vi "FTW-Test-Expressions-Booleanish.vi"() -> (0 "error out":errorcluster)   [LabVIEW 2015]
uses:
  src/error/FTW-ERR-ExceptionType.ctl
  src/expression/FTW-Expr-BooleanExpressionResult.ctl
  src/error/FTW-ERR-ThrowError.vi
  src/error/FTW-ERR-CallChain.vi
  src/error/FTW-ERR-NoErrorConstant.vi
  src/string/FTW-STR-ReplaceWhitespace.vi
  src/string/FTW-STR-Array-Delimit.vi
  src/error/FTW-ERR-Clear.vi
  src/regex/FTW-Regex-ReplaceAll.vi
  lib/FTW-KernelFilepath.vi
panel:
  out "String":string
  out "Array":string[](array[string])
  out "Results":T3(array[cluster])
  out "Lexicon":string="$test == true || $b == false && $c == false"
  out "Capture Groups":string[](array[string])
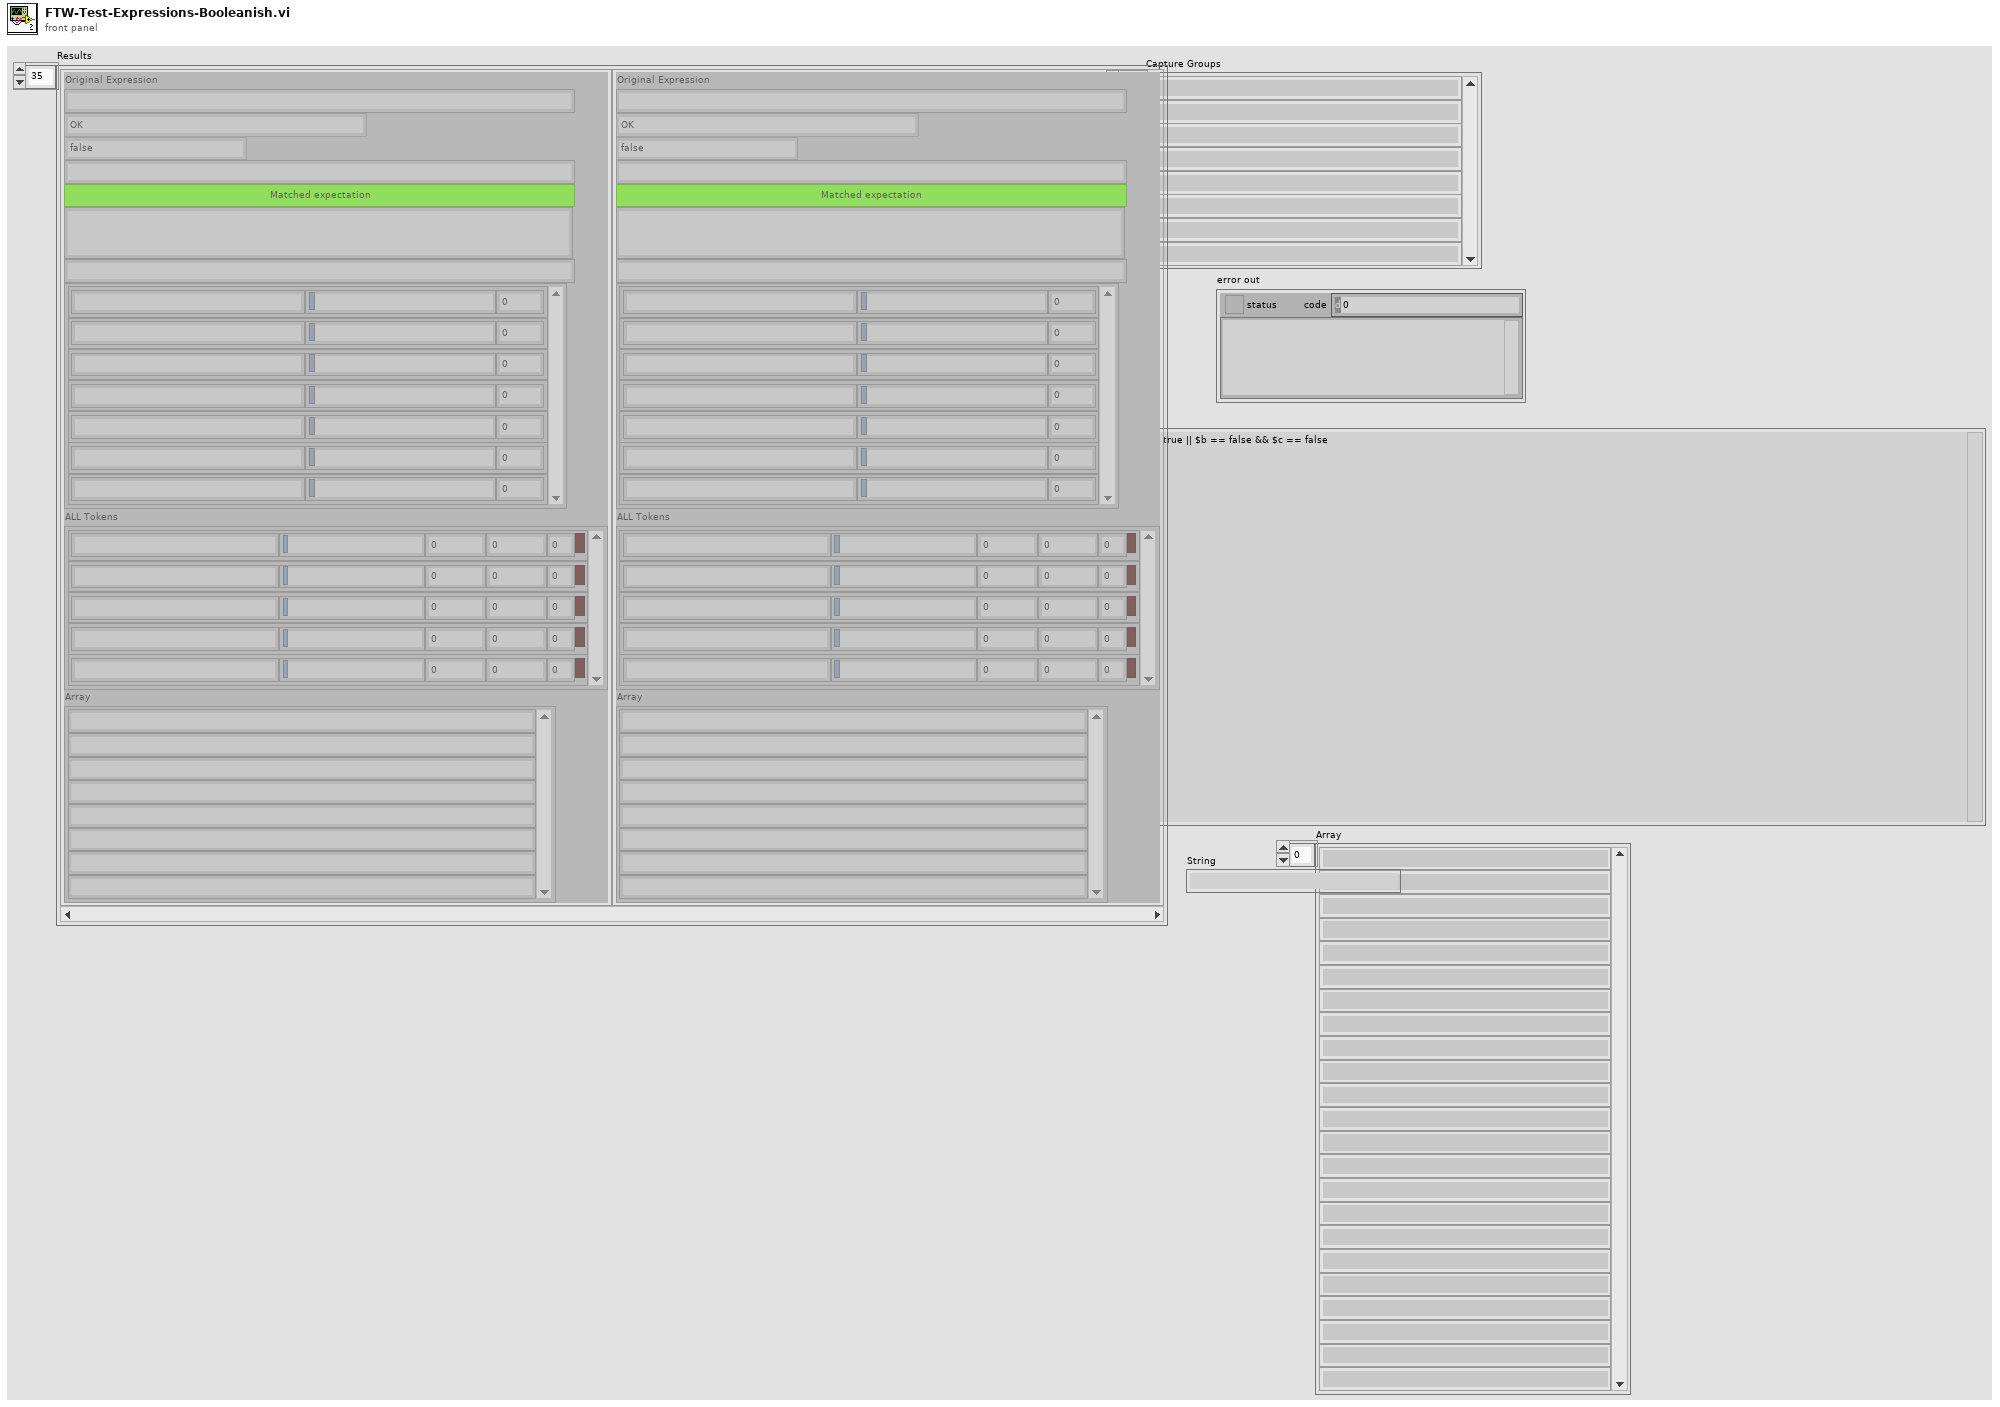
[diagram p1: front panel]
types:
  T1 = typedef "FTW-ERR-ExceptionType.ctl" = enum16{"OK", "Info", "Warning", "Error"}
  T2 = typedef "FTW-Expr-BooleanExpressionResult.ctl" = enum16{"false", "true", "inconclusive"}
  T3 = cluster{"Original Expression":string, "Expression Validity Expectation":T1, "Result":T2, "Expectation":string, "Expectation satisfied?":bool, "Error":string, "Final JSON":string, "Parsed Expression":cluster{string, string, "start_pos":i32}[], "ALL Tokens":cluster{string, string, "prev_pos":i32, "curr_pos":i32, "scope_level":i32, "trimmed?":bool}[], "Array":string[]}[]
  T4 = cluster{"Expression":string, "Expectation":string, "Expression Check":T1, "Value Expectation":T2}[]
  T5 = cluster{"op":cluster{"token":string, "value":string, "subj_start":i32}, "Precedence":i32, "Scope Depth":i32}[]
  T6 = cluster{"token":string, "value":string, "subj_start":i32}[]
  T7 = cluster{"callout_id":i32, "subject_current_pos":i32, "subject_start_match_pos":i32, "cap_top":i32, "cap_last":i32, "patt_pos":i32, "callout_name_index":i32, "callout_name_length":i32}[]
  T8 = cluster{"Text":string, "Expression":string, "Previous Subject Position":i32}
  T9 = cluster{"Text":string, "Expression":string, "Previous Subject Position":i32}[]
  T10 = cluster{cluster{"Text":string, "Expression":string, "Previous Subject Position":i32}, "Precedence":i32, i32}
  T11 = cluster{"op":cluster{"token":string, "value":string, "subj_start":i32}, "Precedence":i32, "Scope Depth":i32}
  T12 = cluster{"token":string, "value":string, "subj_start":i32}
  T13 = cluster{cluster{"Text":string, "Expression":string, "Previous Subject Position":i32}, "default value 1":i32, "Current Scope Depth":i32}
  T14 = cluster{"Text":string, "Expression":string, "subject_current_pos":i32, "Previous Subject Position":i32, "Current Scope Depth":i32, bool}
  T15 = typedef "FTW-JSON-Type.ctl" = enum8{"Not Found", "Object", "Array", "String", "Number", "Boolean", "null"}
  T16 = cluster{"Expression":string, "Expression Check":T1, "Result":T2, "Expectation":string, bool, "source":string, "JSON String (UTF-8)":string, "Reverse Polish Notation Token Stack":cluster{"token":string, "value":string, "subj_start":i32}[], cluster{"Text":string, "Expression":string, "subject_current_pos":i32, "Previous Subject Position":i32, "Current Scope Depth":i32, bool}[], "Try Paths":string[]}
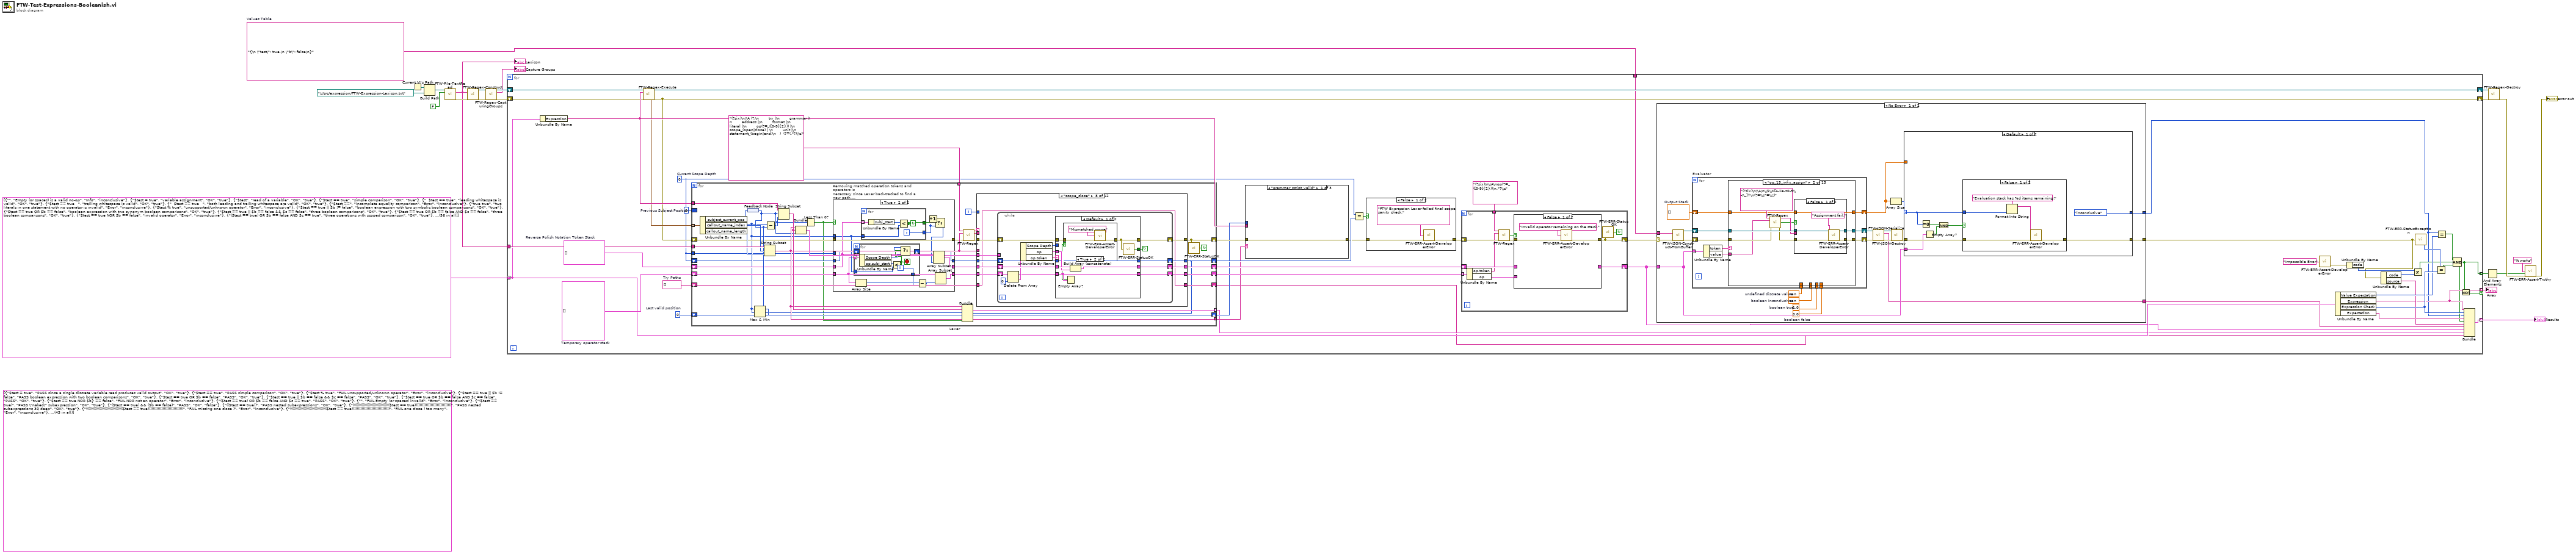
[diagram p0: block diagram]
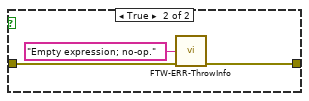
[diagram p2: hidden frame]
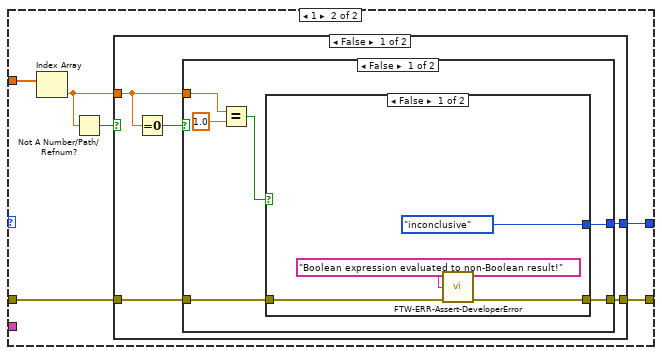
[diagram p3: hidden frame]
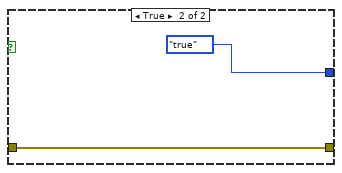
[diagram p4: hidden frame]
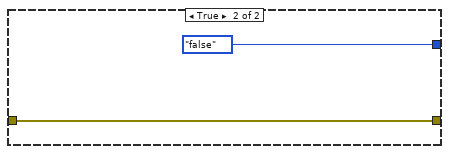
[diagram p5: hidden frame]
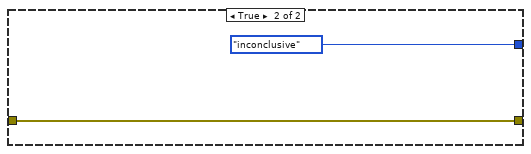
[diagram p6: hidden frame]
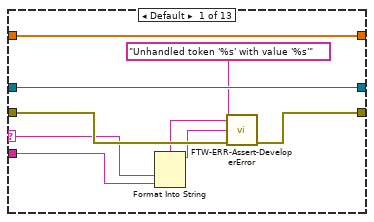
[diagram p7: hidden frame]
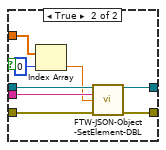
[diagram p8: hidden frame]
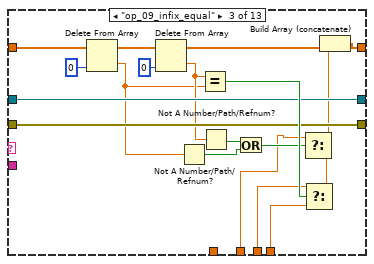
[diagram p9: hidden frame]
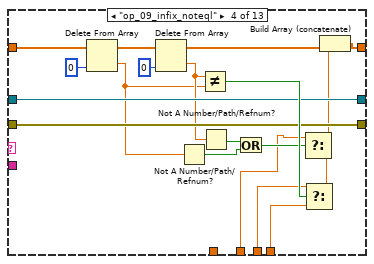
[diagram p10: hidden frame]
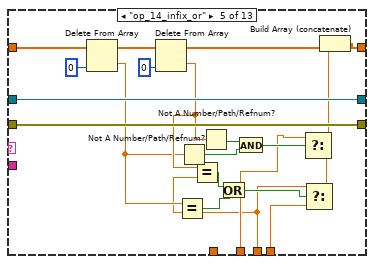
[diagram p11: hidden frame]
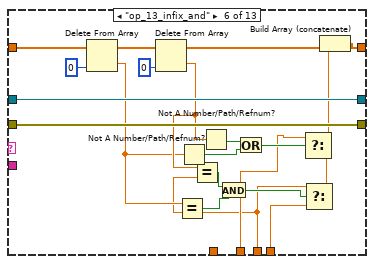
[diagram p12: hidden frame]
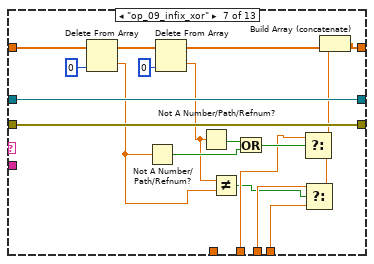
[diagram p13: hidden frame]
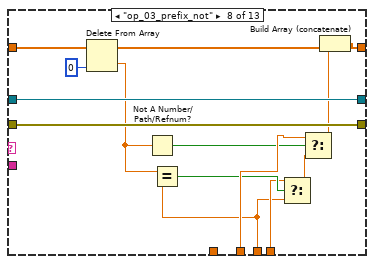
[diagram p14: hidden frame]
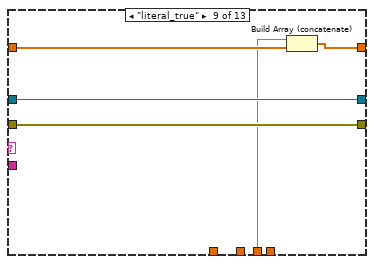
[diagram p15: hidden frame]
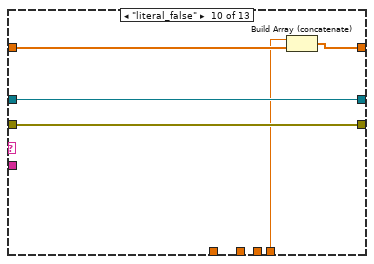
[diagram p16: hidden frame]
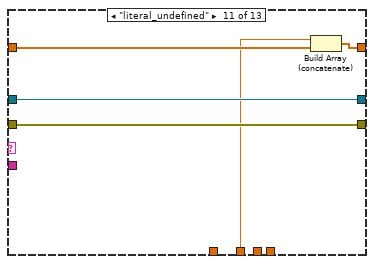
[diagram p17: hidden frame]
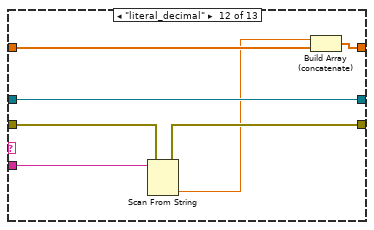
[diagram p18: hidden frame]
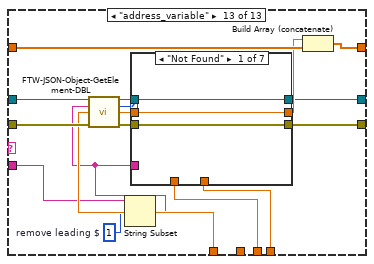
[diagram p19: hidden frame]
diagram:
  (unwired) T4 [{"Expression"="$test = true", "Expectation"="PASS since a single discrete variable read produces valid output", "Expression Check"=enum."OK", "Value Expectation"=enum."true"}, {"Expression"="$test == true", "Expectation"="PASS simple comparison", "Expression Check"=enum."OK", "Value Expectation"=enum."true"}, {"Expression"="$test % true", "Expectation"="FAIL unsupported/unknown operator", "Expression Check"=enum."Error", "Value Expectation"=enum."inconclusive"}, {"Expression"="$test == true || $b != false", "Expectation"="PASS boolean expression with two boolean comparisons", "Expression Check"=enum."OK", "Value Expectation"=enum."true"}, {"Expression"="$test == true OR $b == false", "Expectation"="PASS", "Expression Check"=enum."OK", "Value Expectation"=enum."true"}, {"Expression"="$test == true || $b == false && $c == false", "Expectation"="PASS", "Expression Check"=enum."OK", "Value Expectation"=enum."true"}, {"Expression"="$test == true OR $b == false AND $c == false", "Expectation"="PASS", "Expression Check"=enum."OK", "Value Expectation"=enum."true"}, {"Expression"="$test == true NOR $b} == false", "Expectation"="FAIL NOR not an operator", "Expression Check"=enum."Error", "Value Expectation"=enum."inconclusive"}, {"Expression"="($test == true) OR $b == false AND $c == true", "Expectation"="PASS", "Expression Check"=enum."OK", "Value Expectation"=enum."true"}, {"Expression"="", "Expectation"="FAIL Empty (or spaces) invalid", "Expression Check"=enum."Error", "Value Expectation"=enum."inconclusive"}, {"Expression"="($test == true)", "Expectation"="PASS \"naked\" subexpression", "Expression Check"=enum."OK", "Value Expectation"=enum."true"}, {"Expression"="($test == true) && ($b == false)", "Expectation"="PASS", "Expression Check"=enum."OK", "Value Expectation"=enum."false"}, {"Expression"="(($test == true))", "Expectation"="PASS nested subexpressions", "Expression Check"=enum."OK", "Value Expectation"=enum."true"}, {"Expression"="(((((((((((((((((((((((((((((($test == true))))))))))))))))))))))))))))))", "Expectation"="PASS nested subexpressions 30 deep", "Expression Check"=enum."OK", "Value Expectation"=enum."true"}, {"Expression"="(((((((((((((((((((((((((((((($test == true)))))))))))))))))))))))))))))", "Expectation"="FAIL missing one close )", "Expression Check"=enum."Error", "Value Expectation"=enum."inconclusive"}, {"Expression"="(((((((((((((((((((((((((((((($test == true)))))))))))))))))))))))))))))))", "Expectation"="FAIL one close ) too many", "Expression Check"=enum."Error", "Value Expectation"=enum."inconclusive"}, {"Expression"="true", "Expectation"="PASS plain constant", "Expression Check"=enum."OK", "Value Expectation"=enum."true"}, {"Expression"="False", "Expectation"="PASS plain constant", "Expression Check"=enum."OK", "Value Expectation"=enum."false"}, {"Expression"="ALWAYS AND NEVER", "Expectation"="PASS expression of two boolexpr constants", "Expression Check"=enum."OK", "Value Expectation"=enum."inconclusive"}, {"Expression"="ALWAYS XOR NEVER", "Expectation"="PASS expression of two boolexpr constants", "Expression Check"=enum."OK", "Value Expectation"=enum."inconclusive"}, {"Expression"="(true == true) AND (true EQUALS true) AND (true IS true)", "Expectation"="PASS testing equality operators", "Expression Check"=enum."OK", "Value Expectation"=enum."true"}, {"Expression"="(true != false) AND (true IS NOT false) AND (true <> false)", "Expectation"="PASS testing inequality operators", "Expression Check"=enum."OK", "Value Expectation"=enum."true"}, {"Expression"="(always AND never) XOR (never AND always)", "Expectation"="PASS compound expression of boolexpr constants", "Expression Check"=enum."OK", "Value Expectation"=enum."false"}, {"Expression"="$A==$B", "Expectation"="PASS compare two variables to each other", "Expression Check"=enum."OK", "Value Expectation"=enum."inconclusive"}, {"Expression"="$a!=$b", "Expectation"="PASS since this is a synonym for XOR", "Expression Check"=enum."OK", "Value Expectation"=enum."inconclusive"}, {"Expression"="$A AND $B", "Expectation"="PASS assuming, variables are boolexpr states", "Expression Check"=enum."OK", "Value Expectation"=enum."inconclusive"}, {"Expression"="$a IS true for 3 sec", "Expectation"="SKIP PASS simple timer test", "Expression Check"=enum."OK", "Value Expectation"=enum."inconclusive"}, {"Expression"="$a IS true for 3min", "Expectation"="SKIP PASS no space between timer value and unit", "Expression Check"=enum."OK", "Value Expectation"=enum."inconclusive"}, {"Expression"="$a IS true for 3", "Expectation"="SKIP FAIL no timer units", "Expression Check"=enum."OK", "Value Expectation"=enum."inconclusive"}, {"Expression"="$a IS true   for minute", "Expectation"="SKIP FAIL no timer value", "Expression Check"=enum."OK", "Value Expectation"=enum."inconclusive"}, {"Expression"="$a == true || $b AND $c", "Expectation"="PASS", "Expression Check"=enum."OK", "Value Expectation"=enum."inconclusive"}, {"Expression"="alwaysornever", "Expectation"="FAIL no word boundary on neither operator nor constants", "Expression Check"=enum."OK", "Value Expectation"=enum."inconclusive"}, {"Expression"="always||never", "Expectation"="PASS even though no spaces, the symbolic operator makes a word boundary", "Expression Check"=enum."OK", "Value Expectation"=enum."inconclusive"}, {"Expression"="(($a&&$b) OR ($c&&$d)) AND (($e&&$f) OR ($g&&$h))", "Expectation"="PASS compound expression", "Expression Check"=enum."OK", "Value Expectation"=enum."inconclusive"}, {"Expression"="$a (AND $b)", "Expectation"="FAIL improper placement of parentheses", "Expression Check"=enum."OK", "Value Expectation"=enum."inconclusive"}, {"Expression"="($a)($b)", "Expectation"="FAIL no operator between scopes", "Expression Check"=enum."OK", "Value Expectation"=enum."inconclusive"}, {"Expression"="($a)                   or                 ($b)", "Expectation"="PASS goofy amount of space", "Expression Check"=enum."OK", "Value Expectation"=enum."inconclusive"}, {"Expression"="NOT ALWAYS", "Expectation"="PASS the inversion of a boolexpr constant", "Expression Check"=enum."OK", "Value Expectation"=enum."inconclusive"}, {"Expression"="NOT $a || $b", "Expectation"="PASS even though it could use some parentheses for clarity, this is valid", "Expression Check"=enum."OK", "Value Expectation"=enum."inconclusive"}, {"Expression"="NOT ($a || $b)", "Expectation"="PASS", "Expression Check"=enum."OK", "Value Expectation"=enum."inconclusive"}, {"Expression"="(NOT $a) || $b", "Expectation"="PASS", "Expression Check"=enum."OK", "Value Expectation"=enum."inconclusive"}, {"Expression"="$a && !$b", "Expectation"="PASS", "Expression Check"=enum."OK", "Value Expectation"=enum."inconclusive"}, {"Expression"="IMMEDIATELY", "Expectation"="PASS this is a synonym for ALWAYS", "Expression Check"=enum."OK", "Value Expectation"=enum."inconclusive"}]
  w8 = "{\n \"test\": true,\n \"b\": false\n}"  # Values Table
  n1 = Current VI's Path() -> (path=w18:path)
  n2 = Build Path(base path=w18, name or relative path=path "../../../src/expression/FTW-Expression-Lexicon.txt" ("path")) -> (appended path=w16:path)
  n3 = call "FTW-File-TextRead.vi"("Filepath"=w16, "Create if doesn't exist?"=FALSE) -> ("Text"=w19:string, "error out"=w20:errorcluster)  [unwired: 11 in, 1 out]
  "Lexicon" <- w19
  n4 = call "FTW-Regex-Construct.vi"("Regular Expression"=w19, "error in"=w20) -> ("Regex"=w14:refnum<data-value>, "error out"=w15:errorcluster)  [unwired: 12 in]
  n5 = call "FTW-Regex-CapturingGroups.vi"("Regex"=w14, "error in"=w15) -> ("Regex out"=w22:refnum<data-value>, "Capture Groups"=→"Capture Groups":string[], "error out"=w9:errorcluster)  [unwired: 11 in]
  n6 = for {
    tunnel: w19 -> [w70]
    shift-right: [w55] -> w12
    shift-left: w22 -> [w71]
    tunnel: T4 [{"Expression"="", "Expectation"="Empty (or spaces) is a valid no-op", "Expression Check"=enum."Info", "Value Expectation"=enum."inconclusive"}, {"Expression"="$test = true", "Expectation"="variable assignment", "Expression Check"=enum."OK", "Value Expectation"=enum."true"}, {"Expression"="$test", "Expectation"="read of a variable", "Expression Check"=enum."OK", "Value Expectation"=enum."true"}, {"Expression"="$test == true", "Expectation"="simple comparison", "Expression Check"=enum."OK", "Value Expectation"=enum."true"}, {"Expression"="  $test == true", "Expectation"="leading whitespace is valid", "Expression Check"=enum."OK", "Value Expectation"=enum."true"}, {"Expression"="$test == true   ", "Expectation"="trailing whitespace is valid", "Expression Check"=enum."OK", "Value Expectation"=enum."true"}, {"Expression"="  $test == true   ", "Expectation"="both leading and trailing whitespace are valid", "Expression Check"=enum."OK", "Value Expectation"=enum."true"}, {"Expression"="$test ==", "Expectation"="incomplete equality comparison", "Expression Check"=enum."Error", "Value Expectation"=enum."inconclusive"}, {"Expression"="true true", "Expectation"="two literals in one statement with no operator is invalid", "Expression Check"=enum."Error", "Value Expectation"=enum."inconclusive"}, {"Expression"="$test % true", "Expectation"="unsupported/unknown operator", "Expression Check"=enum."Error", "Value Expectation"=enum."inconclusive"}, {"Expression"="$test == true || $b != false", "Expectation"="boolean expression with two symbolic boolean comparisons", "Expression Check"=enum."OK", "Value Expectation"=enum."true"}, {"Expression"="$test == true OR $b == false", "Expectation"="boolean expression with two synonym boolean comparisons", "Expression Check"=enum."OK", "Value Expectation"=enum."true"}, {"Expression"="$test == true || $b == false && $c == false", "Expectation"="three boolean comparisons", "Expression Check"=enum."OK", "Value Expectation"=enum."true"}, {"Expression"="$test == true OR $b == false AND $c == false", "Expectation"="three boolean comparisons", "Expression Check"=enum."OK", "Value Expectation"=enum."true"}, {"Expression"="$test == true NOR $b == false", "Expectation"="invalid operator", "Expression Check"=enum."Error", "Value Expectation"=enum."inconclusive"}, {"Expression"="($test == true) OR $b == false AND $c == true", "Expectation"="three operations with scoped comparison", "Expression Check"=enum."OK", "Value Expectation"=enum."true"}, {"Expression"="$test OR ($test == false)", "Expectation"="variable comparison with subexpression", "Expression Check"=enum."OK", "Value Expectation"=enum."true"}, {"Expression"="($test == true)", "Expectation"="superfluous subexpression", "Expression Check"=enum."OK", "Value Expectation"=enum."true"}, {"Expression"="($test == true) && ($b == false)", "Expectation"="operation on two subexpressions", "Expression Check"=enum."OK", "Value Expectation"=enum."true"}, {"Expression"="(($test == true))", "Expectation"="nested subexpressions", "Expression Check"=enum."OK", "Value Expectation"=enum."true"}, {"Expression"="(((((((((((((((((((((((((((((($test == true))))))))))))))))))))))))))))))", "Expectation"="PASS nested subexpressions 30 deep", "Expression Check"=enum."OK", "Value Expectation"=enum."true"}, {"Expression"="(((((((((((((((((((((((((((((($test == true)))))))))))))))))))))))))))))", "Expectation"="missing one close )", "Expression Check"=enum."Error", "Value Expectation"=enum."inconclusive"}, {"Expression"="(((((((((((((((((((((((((((((($test == true)))))))))))))))))))))))))))))))", "Expectation"="one close ) too many", "Expression Check"=enum."Error", "Value Expectation"=enum."inconclusive"}, {"Expression"="true", "Expectation"="plain constant", "Expression Check"=enum."OK", "Value Expectation"=enum."true"}, {"Expression"="False", "Expectation"="plain constant", "Expression Check"=enum."OK", "Value Expectation"=enum."false"}, {"Expression"="true XOR false", "Expectation"="expression of two boolexpr constants", "Expression Check"=enum."OK", "Value Expectation"=enum."true"}, {"Expression"="(true == true) AND (true EQUALS true) AND (true IS true)", "Expectation"="testing equality operators", "Expression Check"=enum."OK", "Value Expectation"=enum."true"}, {"Expression"="(true != false) AND (true IS NOT false) AND (true <> false)", "Expectation"="testing inequality operators", "Expression Check"=enum."OK", "Value Expectation"=enum."true"}, {"Expression"="(true AND false) XOR (false AND true)", "Expectation"="compound expression of boolexpr constants", "Expression Check"=enum."OK", "Value Expectation"=enum."false"}, {"Expression"="$A==$B", "Expectation"="compare two variables to each other", "Expression Check"=enum."OK", "Value Expectation"=enum."inconclusive"}, {"Expression"="$a!=$b", "Expectation"="synonym for XOR", "Expression Check"=enum."OK", "Value Expectation"=enum."inconclusive"}, {"Expression"="$A AND $B", "Expectation"="AND two variables", "Expression Check"=enum."OK", "Value Expectation"=enum."inconclusive"}, {"Expression"="$test == ture", "Expectation"="common misspelling of \"true\" is invalid", "Expression Check"=enum."Error", "Value Expectation"=enum."inconclusive"}, {"Expression"="%test == flase", "Expectation"="common misspelling of \"false\" is invalid", "Expression Check"=enum."Error", "Value Expectation"=enum."inconclusive"}, {"Expression"="$test == tru", "Expectation"="incomplete literal \"true\"", "Expression Check"=enum."Error", "Value Expectation"=enum."inconclusive"}, {"Expression"="$test == truee", "Expectation"="extra 'e' in literal \"true\"", "Expression Check"=enum."Error", "Value Expectation"=enum."inconclusive"}, {"Expression"="$test == true!", "Expectation"="unary operator in wrong location", "Expression Check"=enum."Error", "Value Expectation"=enum."inconclusive"}, {"Expression"="$a == true || $b AND $c", "Expectation"="mix of symbolic and synonym operators", "Expression Check"=enum."OK", "Value Expectation"=enum."inconclusive"}, {"Expression"="falseortrue", "Expectation"="invalid without word boundary between operator and literals", "Expression Check"=enum."Error", "Value Expectation"=enum."inconclusive"}, {"Expression"="false||true", "Expectation"="even though no spaces, the symbolic operator makes a word boundary", "Expression Check"=enum."OK", "Value Expectation"=enum."true"}, {"Expression"="(($a&&$b) OR ($c&&$d)) AND (($e&&$f) OR ($g&&$h))", "Expectation"="compound scoped expression", "Expression Check"=enum."OK", "Value Expectation"=enum."inconclusive"}, {"Expression"="$a (AND $b)", "Expectation"="improper placement of parentheses", "Expression Check"=enum."Error", "Value Expectation"=enum."inconclusive"}, {"Expression"="($a)($b)", "Expectation"="no operator between scopes", "Expression Check"=enum."Error", "Value Expectation"=enum."inconclusive"}, {"Expression"="($a)                   or                 ($b)", "Expectation"="goofy but valid amount of space", "Expression Check"=enum."OK", "Value Expectation"=enum."false"}, {"Expression"="NOT $a || $b", "Expectation"="valid, but could use some parentheses for clarity, since precedence applies to first operand and not the result of the operation", "Expression Check"=enum."OK", "Value Expectation"=enum."false"}, {"Expression"="$b || NOT $a", "Expectation"="valid", "Expression Check"=enum."OK", "Value Expectation"=enum."false"}, {"Expression"="$b||!$a", "Expectation"="could use some whitespace, but valid use of symbolic operators", "Expression Check"=enum."OK", "Value Expectation"=enum."false"}, {"Expression"="NOT ($a || $b)", "Expectation"="valid", "Expression Check"=enum."OK", "Value Expectation"=enum."true"}, {"Expression"="(NOT $a) || $b", "Expectation"="valid", "Expression Check"=enum."OK", "Value Expectation"=enum."false"}, {"Expression"="!($a||$b)", "Expectation"="valid", "Expression Check"=enum."OK", "Value Expectation"=enum."true"}, {"Expression"="$a && !$b", "Expectation"="valid", "Expression Check"=enum."OK", "Value Expectation"=enum."inconclusive"}, {"Expression"="! ($test = false)", "Expectation"="assignment in the middle of a statement", "Expression Check"=enum."OK", "Value Expectation"=enum."true"}, {"Expression"="$b | true", "Expectation"="unsupported operator `|`", "Expression Check"=enum."Error", "Value Expectation"=enum."inconclusive"}, {"Expression"="$b & true", "Expectation"="unsupported operator `&`", "Expression Check"=enum."Error", "Value Expectation"=enum."inconclusive"}, {"Expression"="$b IS NOT true", "Expectation"="inequality on boolean", "Expression Check"=enum."OK", "Value Expectation"=enum."true"}, {"Expression"="$b IS NOT NOT false", "Expectation"="inequality on inverted boolean", "Expression Check"=enum."OK", "Value Expectation"=enum."true"}] -> [w53] mode=indexing
    tunnel: [w54] -> w11 mode=indexing
    tunnel: [w32] -> w10 mode=indexing
    tunnel: w8 -> [w42]
    shift-right: [w40] -> w7
    shift-left: w9 -> [w44]
    tunnel: [w33] -> w6 mode=indexing if=w31
    w28 = 0  # Previous Subject Position
    w30 = string[] []  # Try Paths
    w58 = 0  # Last valid position
    w24 = 0  # Current Scope Depth
    w67 = T5 []  # Temporary operator stack
    w68 = T6 []  # Reverse Polish Notation Token Stack
    n7 = Unbundle By Name(w53) -> ("Expression"=w52:string)
    n8 = call "FTW-Regex-Execute.vi"("Regex"=w71, "Subject String"=w52, "error in"=w44) -> ("Regex out"=w55:refnum<data-value>, "Callouts"=w41:T7, "error out"=w40:errorcluster)  [unwired: 7 in, 3 out]
    n9 = for "Lexer" {
      tunnel: "(?six)\n\\A (?:\n        try |\n        grammar |\n        address |\n        format |\n        literal |\n        op(?=_([0-9]{2})) |\n        scope_(open|close) | \n        unit |\n        statement_(begin|end)\n   )  (?=(.*?)\\z)" -> [w429]
      shift-right: [w426] -> w59
      shift-left: w68 -> [w404]
      shift-right: [w424] -> w61
      shift-left: w40 -> [w402]
      shift-right: [w422] -> w66
      shift-left: w67 -> [w405]
      shift-right: [w394] -> w64
      shift-left: w24 -> [w398]
      tunnel: w41 -> [w419] mode=indexing
      tunnel: w52 -> [w421]
      tunnel: [w412] -> w43 mode=indexing
      shift-right: [w417] -> w57
      shift-left: w58 -> [w418]
      tunnel: [w410] -> w56
      tunnel: w70 -> [w416]
      shift-right: [w408] -> w29
      shift-left: w30 -> [w409]
      border: w28 -> [_]
      tunnel: w24 -> [w396]
      i -> [w420]
      stop <- w423 continue-if-true
      n10 = Unbundle By Name(w419) -> ("subject_current_pos"=w399:i32, "callout_name_index"=w415:i32, "callout_name_length"=w414:i32)
      n11 = feedback-in #1(w399) -> ()
      n12 = feedback #1() -> (w407:i32)
      n13 = Max & Min(x=w399, y=w418) -> (max(x,y)=w417:i32)  [unwired: 1 out]
      n14 = String Subset(string=w416, offset (0)=w415, length (rest)=w414) -> (substring=w410:string)
      n15 = Subtract(x=w399, y=w407) -> (x-y=w406:i32)
      n16 = String Subset(string=w421, offset (0)=w407, length (rest)=w406) -> (substring=w411:string)
      n17 = Bundle("Text"=w410, "Expression"=w411, "Previous Subject Position"=w407) -> (w413:T8)  [unwired: 1 in]
      n18 = Less Than 0?(x=w406) -> (x < 0?=w395:bool)
      n19 = case "Removing matched operation tokens and operators is \nnecessary since Lexer back-tracked to find a new path,\nnot having found complete grammar of a valid expression" shown="True" w395 {
        tunnel: w405 -> [w432 w437]
        tunnel: w404 -> [w433 w447]
        tunnel: [w431 w448] -> w403
        tunnel: w402 -> [w431 w448]
        tunnel: [w433 w446] -> w401
        tunnel: [w432 w445] -> w400
        tunnel: w399 -> [_ w444]
        tunnel: w398 -> [w430 w438]
        tunnel: [w430 w443] -> w397
        tunnel: w396 -> [_ _]
        frame False {
        }
        frame True {
          n20 = for {
            tunnel: w437 -> [w456] mode=indexing
            tunnel: w444 -> [w454]
            shift-right: [w451] -> w443
            shift-left: w438 -> [w452]
            tunnel: [w449] -> w434
            i -> [w449]
            stop <- w450 stop-if-true
            n21 = Unbundle By Name(w456) -> ("Scope Depth"=w453:i32, "op.subj_start"=w455:i32)
            n22 = Less?(x=w455, y=w454) -> (x < y?=w450:bool)
            n23 = Select(t=w452, s=w450, f=w453) -> (s? t:f=w451:i32)
          }
          n24 = Array Size(array=w437) -> (size(s)=w436:i32)
          n25 = for {
            tunnel: w447 -> [w461] mode=indexing
            tunnel: w444 -> [w459]
            tunnel: [w458] -> w440
            tunnel: [w457] -> w442
            i -> [w458]
            stop <- w457 continue-if-true
            n26 = Unbundle By Name(w461) -> ("subj_start"=w460:i32)
            n27 = Less?(x=w460, y=w459) -> (x < y?=w457:bool)
          }
          n28 = Subtract(x=w436, y=w434) -> (x-y=w435:i32)
          n29 = Increment(x=w440) -> (x+1=w439:i32)
          n30 = Select(t=w439, s=w442, f=w440) -> (s? t:f=w441:i32)
          n31 = Array Subset(array=w447, length=w441) -> (w446:T6)  [unwired: 1 in]
          n32 = Array Subset(array=w437, length=w435) -> (w445:T5)  [unwired: 1 in]
        }
      }
      n33 = call "FTW-Regex.vi"("Regular Expression"=w429, "Input String"=w410, "error in"=w403) -> ("Match"=w428:string, "Submatches"=w427:string[], "error out"=w425:errorcluster)  [unwired: 8 in, 2 out]
      n34 = case shown="\"scope_close\"" w428 {
        tunnel: w427 -> [_ _ _ _ w494 _ _ _ w569 _ _ _]
        tunnel: w413 -> [_ w477 w484 _ _ _ w511 w521 w570 _ _ _]
        tunnel: w401 -> [w468 w476 w483 w489 w498 w505 w514 w525 w574 w630 w635 w640]
        tunnel: [w468 w475 w482 w489 w498 w505 w514 w523 w575 w630 w635 w640] -> w426
        tunnel: [w469 w474 w481 w488 w497 w502 w515 w520 w572 w631 w636 w641] -> w424
        tunnel: w425 -> [w470 w474 w481 w488 w497 w502 w515 w519 w579 w631 w636 w641]
        tunnel: [w467 w473 w480 w487 w496 w504 w512 w522 w571 w629 w634 w639] -> w422
        tunnel: w400 -> [w467 w473 w480 w487 w496 w504 w513 w524 w576 w629 w634 w639]
        tunnel: w410 -> [w464 _ _ _ w490 w499 _ _ _ _ _ _]
        tunnel: w397 -> [w463 w472 w479 w486 w495 w503 w509 w518 w567 w628 w633 w638]
        tunnel: [w463 w472 w479 w486 w495 w503 w508 w517 w567 w628 w633 w638] -> w394
        tunnel: w420 -> [_ _ _ _ _ _ _ _ _ _ _ _]
        tunnel: w409 -> [w462 w471 w478 w485 w492 w501 w506 w516 w566 w627 w632 w637]
        tunnel: [w462 w471 w478 w485 w491 w500 w506 w516 w566 w627 w632 w637] -> w408
        frame Default {
          n35 = Format Into String(format string="Bug in the FTW evaluation compiler! Unknown token: \"%s\"" ("Reason this error should never happen"), w464) -> (resulting string=w465:string)  [unwired: 2 in, 1 out]
          n36 = call "FTW-ERR-Assert-DeveloperError.vi"("Reason this error should never happen"=w465, "error in"=w470) -> ("error out"=w469:errorcluster)  [unwired: 13 in]
        }
        frame "literal" {
          n37 = Build Array (concatenate)(w476, w477) -> (w475:T9)
        }
        frame "address" {
          n38 = Build Array (concatenate)(w483, w484) -> (w482:T9)
        }
        frame "format" {
          # "Format matches are included in the\ncallout array purely to maintain match position\nof tokens."
        }
        frame "try" {
          # "Format matches are included in the\ncallout array purely to maintain match position\nof tokens."
          n39 = Index Array(array=w494) -> (element=→"String":string)  [unwired: 1 in]
          n40 = Build Array (concatenate)(w492, w490) -> (w491:string[])
        }
        frame "grammar" {
          # "Grammar matches are included in the\ncallout array in order to maintain match position\nof tokens and to validate grammar."
          n41 = Build Array (concatenate)(w501, w499) -> (w500:string[])
        }
        frame "scope_open" {
          w507 = -1  # Precedence
          n42 = Increment(x=w509) -> (x+1=w508:i32)
          n43 = Bundle(w511, "Precedence"=w507, w508) -> (w510:T10)  [unwired: 1 in]
          n44 = Build Array (concatenate)(w510, w513) -> (w512:T5)
        }
        frame "scope_close" {
          n45 = while {
            shift-right: [w531] -> w520
            shift-left: w519 -> [w532]
            shift-right: [w540] -> w523
            shift-left: w525 -> [w539]
            shift-right: [w538] -> w522
            shift-left: w524 -> [w537]
            tunnel: w521 -> [_]
            shift-right: [w528] -> w517
            shift-left: w518 -> [w527]
            stop <- w529 continue-if-true
            n46 = Delete From Array(array=w537, index=0) -> (deleted portion=w535:T11, array with subset deleted=w533:T5)  [unwired: 1 in]
            n47 = Unbundle By Name(w535) -> ("Scope Depth"=w526:i32, "op"=w530:T12, "op.token"=w534:string)
            n48 = case shown="Default" w534 {
              tunnel: [w549 w561] -> w540
              tunnel: w539 -> [w548 w561]
              tunnel: [w545 w560] -> w538
              tunnel: w533 -> [w545 w560]
              tunnel: w532 -> [w546 w556]
              tunnel: [w543 w555] -> w531
              tunnel: w530 -> [w547 _]
              tunnel: [w542 _] -> w529
              tunnel: [w541 w559] -> w528
              tunnel: w527 -> [w541 w557]
              tunnel: w526 -> [_ w558]
              frame Default {
                n49 = Empty Array?(array=w545) -> (empty?=w544:bool)
                n50 = case shown="True" w544 {
                  tunnel: w546 -> [w550 w553]
                  tunnel: [w550 w551] -> w543
                  frame False {
                  }
                  frame True {
                    n51 = call "FTW-ERR-Assert-DeveloperError.vi"("Reason this error should never happen"="Mismatched scope", "error in"=w553) -> ("error out"=w551:errorcluster)  [unwired: 13 in]
                  }
                }
                n52 = Build Array (concatenate)(w548, w547) -> (w549:T6)
                n53 = call "FTW-ERR-StatusOK.vi"("error to check"=w543) -> ("Status OK?"=w542:bool)
              }
              frame "scope_open" {
                # "Found it the matching\nscope_open token;\nsilently discard it."
                n54 = Not Equal?(x=w558, y=w557) -> (x != y?=w554:bool)
                n55 = case shown="True" w554 {
                  tunnel: w556 -> [w562 w565]
                  tunnel: [w562 w563] -> w555
                  frame False {
                  }
                  frame True {
                    n56 = call "FTW-ERR-Assert-DeveloperError.vi"("Reason this error should never happen"="Mismatched scope level", "error in"=w565) -> ("error out"=w563:errorcluster)  [unwired: 13 in]
                  }
                }
                n57 = Decrement(x=w557) -> (x-1=w559:i32)
              }
            }
          }
        }
        frame "op" {
          n58 = Index Array(array=w569) -> (element=w568:string)  [unwired: 1 in]
          n59 = Scan From String(input string=w568, error in=w579, default 1=-1 ("default value 1")) -> (error out=w573:errorcluster, output 1=w577:i32)  [unwired: 2 in, 2 out]
          n60 = while {
            tunnel: w577 -> [w585]
            shift-right: [w581] -> w572
            shift-left: w573 -> [w580]
            shift-right: [w590] -> w575
            shift-left: w574 -> [w589]
            shift-right: [w588] -> w571
            shift-left: w576 -> [w587]
            tunnel: w570 -> [w586]
            tunnel: w567 -> [w584]
            stop <- w582 continue-if-true
            n61 = Empty Array?(array=w587) -> (empty?=w583:bool)
            n62 = case shown="False" w583 {
              tunnel: [w599 w612] -> w590
              tunnel: w589 -> [w599 w611]
              tunnel: [w598 w610] -> w588
              tunnel: w587 -> [w597 w606]
              tunnel: w586 -> [w596 w609]
              tunnel: w585 -> [w595 w608]
              tunnel: w584 -> [w594 w607]
              tunnel: [FALSE w600] -> w582
              tunnel: [w591 w604] -> w581
              tunnel: w580 -> [w591 w604]
              frame True {
                n63 = Bundle(w596, "default value 1"=w595, "Current Scope Depth"=w594) -> (w593:T13)  [unwired: 1 in]
                n64 = Build Array (concatenate)(w593, w597) -> (w598:T5)
              }
              frame False {
                n65 = Index Array(array=w606) -> (element=w605:T11)  [unwired: 1 in]
                n66 = Unbundle By Name(w605) -> ("Precedence"=w603:i32)
                n67 = Greater Or Equal?(x=w608, y=w603) -> (x >= y?=w602:bool)
                n68 = Greater Or Equal To 0?(x=w603) -> (x >= 0?=w601:bool)
                n69 = And(x=w602, y=w601) -> (x .and. y?=w600:bool)
                n70 = case shown="False" w600 {
                  tunnel: [w619 w625] -> w612
                  tunnel: w611 -> [w619 w626]
                  tunnel: [w617 w620] -> w610
                  tunnel: w606 -> [w618 w621]
                  tunnel: w609 -> [w616 _]
                  tunnel: w608 -> [w615 _]
                  tunnel: w607 -> [w613 _]
                  frame False {
                    n71 = Bundle(w616, "default value 1"=w615, "Current Scope Depth"=w613) -> (w614:T13)  [unwired: 1 in]
                    n72 = Build Array (concatenate)(w614, w618) -> (w617:T5)
                  }
                  frame True {
                    n73 = Delete From Array(array=w621, index=0) -> (deleted portion=w623:T11, array with subset deleted=w620:T5)  [unwired: 1 in]
                    n74 = Unbundle(w623) -> ("op"=w622:T12)  [unwired: 2 out]
                    n75 = Build Array (concatenate)(w626, w622) -> (w625:T6)
                  }
                }
              }
            }
          }
        }
        frame "unit" {
        }
        frame "statement_begin" {
        }
        frame "statement_end" {
        }
      }
      n76 = Bundle("Text"=w410, "Expression"=w411, "subject_current_pos"=w399, "Previous Subject Position"=w407, "Current Scope Depth"=w394, w395) -> (w412:T14)  [unwired: 1 in]
      n77 = call "FTW-ERR-StatusOK.vi"("error to check"=w424) -> ("Status OK?"=w423:bool)
    }
    n78 = case shown="\"grammar_script_valid\"" w56 {
      tunnel: [w360 w362 w371] -> w60
      tunnel: w61 -> [w360 w363 w370]
      tunnel: w57 -> [_ _ w366]
      tunnel: w52 -> [_ _ w367]
      frame "grammar_script_valid" {
      }
      frame Default {
        n79 = call "FTW-ERR-Assert-DeveloperError.vi"("Reason this error should never happen"="Bogus lexing regex.", "error in"=w363) -> ("error out"=w362:errorcluster)  [unwired: 13 in]
      }
      frame "grammar_script_invalid" {
        n80 = String Subset(string=w367, offset (0)=w366, length (rest)=8 ("length (rest)")) -> (substring=w364:string)
        n81 = Format Into String(format string="Syntax error near character position %d beginning with \"%s\"" ("Error Message"), w366, w364) -> (resulting string=w368:string)  [unwired: 2 in, 1 out]
        n82 = call "FTW-ERR-ThrowGenericError.vi"("Error Message"=w368, "error in"=w370) -> ("error out"=w371:errorcluster)  [unwired: 13 in]
      }
    }
    n83 = Equal?(x=w24, y=w64) -> (x = y?=w63:bool)
    n84 = case shown="False" w63 {
      tunnel: w60 -> [w373 w375]
      tunnel: [w372 w375] -> w62
      frame False {
        n85 = call "FTW-ERR-Assert-DeveloperError.vi"("Reason this error should never happen"="FTW Expression Lexer failed final scope sanity check.", "error in"=w373) -> ("error out"=w372:errorcluster)  [unwired: 13 in]
      }
      frame True {
      }
    }
    n86 = for {
      tunnel: w66 -> [w386] mode=indexing
      shift-right: [w377] -> w34
      shift-left: w62 -> [w385]
      tunnel: "(?six)\n\\A\nop(?=_([0-9]{2}))\n.*?\\z" ("Regular Expression") -> [w384]
      shift-right: [w379] -> w26
      shift-left: w59 -> [w380]
      stop <- w376 continue-if-true
      n87 = Unbundle By Name(w386) -> ("op.token"=w378:string, "op"=w381:T12)
      n88 = call "FTW-Regex.vi"("Regular Expression"=w384, "Input String"=w378, "error in"=w385) -> ("Match Found?"=w383:bool, "error out"=w382:errorcluster)  [unwired: 8 in, 3 out]
      n89 = case shown="False" w383 {
        tunnel: w382 -> [w389 w393]
        tunnel: [w387 w393] -> w377
        tunnel: w381 -> [_ w392]
        tunnel: w380 -> [_ w391]
        tunnel: [_ w390] -> w379
        frame False {
          n90 = call "FTW-ERR-Assert-DeveloperError.vi"("Reason this error should never happen"="Invalid operator remaining on the stack.", "error in"=w389) -> ("error out"=w387:errorcluster)  [unwired: 13 in]
        }
        frame True {
          n91 = Build Array (concatenate)(w391, w392) -> (w390:T6)
        }
      }
      n92 = call "FTW-ERR-StatusOK.vi"("error to check"=w377) -> ("Status OK?"=w376:bool)
    }
    n93 = case shown="No Error" w34 {
      selector: w34 -> [w83 w359]
      tunnel: [w79 w359] -> w25
      tunnel: w26 -> [w77 _]
      tunnel: w42 -> [w84 _]
      tunnel: [w78 FTW-Expr-BooleanExpressionResult."inconclusive" ("Result")] -> w27
      tunnel: [w72 "" ("JSON String (UTF-8)")] -> w23
      frame No Error {
        w85 = nan  # undefined discrete value
        w86 = nan  # boolean inconclusive
        w87 = 1.0  # boolean true
        w88 = 0.0  # boolean false
        w89 = dbl[] []  # Output Stack
        n94 = call "FTW-JSON-Construct-FromBuffer.vi"("JSON String (UTF-8)"=w84, "error in"=w83) -> ("JSON Object"=w90:refnum<data-value>, "error out"=w91:errorcluster)  [unwired: 12 in]
        n95 = for "Evaluator" {
          tunnel: w77 -> [w147] mode=indexing
          shift-right: [w144] -> w81
          shift-left: w89 -> [w145]
          shift-right: [w142] -> w76
          shift-left: w90 -> [w143]
          shift-right: [w140] -> w74
          shift-left: w91 -> [w141]
          tunnel: w88 -> [w139]
          tunnel: w87 -> [w138]
          tunnel: w86 -> [w137]
          tunnel: w85 -> [w136]
          n96 = Unbundle By Name(w147) -> ("token"=w146:string, "value"=w135:string)
          n97 = case shown="\"op_15_infix_assign\"" w146 {
            selector: w146 -> [w149 _ _ _ _ _ _ _ _ _ _ _ _]
            tunnel: w145 -> [w155 w157 w196 w215 w236 w257 w276 w290 w295 w300 w305 w312 w329]
            tunnel: [w155 w157 w190 w209 w231 w252 w271 w288 w294 w299 w304 w311 w328] -> w144
            tunnel: w143 -> [w154 w165 w189 w208 w230 w251 w270 w287 w293 w298 w303 w310 w327]
            tunnel: [w154 w164 w189 w208 w230 w251 w270 w287 w293 w298 w303 w310 w319] -> w142
            tunnel: w141 -> [w153 w162 w188 w207 w229 w250 w269 w286 w292 w297 w302 w308 w326]
            tunnel: [w152 w163 w188 w207 w229 w250 w269 w286 w292 w297 w302 w307 w318] -> w140
            tunnel: w135 -> [w148 w159 _ _ _ _ _ _ _ _ _ w309 w314]
            tunnel: w139 -> [_ _ w180 w199 w223 w244 w263 w279 _ w296 _ _ w316]
            tunnel: w138 -> [_ _ w179 w198 w218 w239 w261 w278 w291 _ _ _ w317]
            tunnel: w137 -> [_ _ w178 w197 w222 w243 w262 w284 _ _ w301 _ _]
            tunnel: w136 -> [_ _ _ _ _ _ _ _ _ _ _ _ w325]
            frame Default {
              n98 = Format Into String(format string="Unhandled token '%s' with value '%s'" ("Reason this error should never happen"), w149, w148) -> (resulting string=w151:string)  [unwired: 2 in, 1 out]
              n99 = call "FTW-ERR-Assert-DeveloperError.vi"("Reason this error should never happen"=w151, "error in"=w153) -> ("error out"=w152:errorcluster)  [unwired: 13 in]
            }
            frame "op_15_infix_assign" {
              n100 = call "FTW-Regex.vi"("Regular Expression"="(?six)\n\\A\n\\$\\K[A-Za-z0-9\\-\\_]+\n(?=\\s*=\\z)", "Input String"=w159, "error in"=w162) -> ("Match"=w158:string, "Match Found?"=w156:bool, "error out"=w161:errorcluster)  [unwired: 8 in, 2 out]
              n101 = case shown="False" w156 {
                tunnel: w165 -> [w169 w177]
                tunnel: [w169 w176] -> w164
                tunnel: [w167 w175] -> w163
                tunnel: w161 -> [w168 w174]
                tunnel: w158 -> [_ w173]
                tunnel: w157 -> [_ w171]
                frame False {
                  n102 = call "FTW-ERR-Assert-DeveloperError.vi"("Reason this error should never happen"="Assignment fail.", "error in"=w168) -> ("error out"=w167:errorcluster)  [unwired: 13 in]
                }
                frame True {
                  n103 = Index Array(array=w171, index=0) -> (element=w170:dbl)
                  n104 = call "FTW-JSON-Object-SetElement-DBL.vi"("JSON Object"=w177, "Key"=w173, "Value"=w170, "error in"=w174) -> ("JSON Object out"=w176:refnum<data-value>, "error out"=w175:errorcluster)  [unwired: 10 in]
                }
              }
            }
            frame "op_09_infix_equal" {
              n105 = Delete From Array(array=w196, index=0) -> (deleted portion=w186:dbl, array with subset deleted=w194:dbl[])  [unwired: 1 in]
              n106 = Delete From Array(array=w194, index=0) -> (deleted portion=w187:dbl, array with subset deleted=w191:dbl[])  [unwired: 1 in]
              n107 = Not A Number/Path/Refnum?(number/path/refnum=w186) -> (NaN/Path/Refnum?=w184:bool)
              n108 = Equal?(x=w187, y=w186) -> (x = y?=w192:bool)
              n109 = Not A Number/Path/Refnum?(number/path/refnum=w187) -> (NaN/Path/Refnum?=w185:bool)
              n110 = Or(x=w185, y=w184) -> (x .or. y?=w183:bool)
              n111 = Select(t=w179, s=w192, f=w180) -> (s? t:f=w182:dbl)
              n112 = Select(t=w178, s=w183, f=w182) -> (s? t:f=w181:dbl)
              n113 = Build Array (concatenate)(w181, w191) -> (w190:dbl[])
            }
            frame "op_09_infix_noteql" {
              n114 = Delete From Array(array=w215, index=0) -> (deleted portion=w205:dbl, array with subset deleted=w213:dbl[])  [unwired: 1 in]
              n115 = Delete From Array(array=w213, index=0) -> (deleted portion=w206:dbl, array with subset deleted=w210:dbl[])  [unwired: 1 in]
              n116 = Not A Number/Path/Refnum?(number/path/refnum=w205) -> (NaN/Path/Refnum?=w203:bool)
              n117 = Not Equal?(x=w206, y=w205) -> (x != y?=w211:bool)
              n118 = Not A Number/Path/Refnum?(number/path/refnum=w206) -> (NaN/Path/Refnum?=w204:bool)
              n119 = Or(x=w204, y=w203) -> (x .or. y?=w202:bool)
              n120 = Select(t=w198, s=w211, f=w199) -> (s? t:f=w201:dbl)
              n121 = Select(t=w197, s=w202, f=w201) -> (s? t:f=w200:dbl)
              n122 = Build Array (concatenate)(w200, w210) -> (w209:dbl[])
            }
            frame "op_14_infix_or" {
              n123 = Delete From Array(array=w236, index=0) -> (deleted portion=w219:dbl, array with subset deleted=w234:dbl[])  [unwired: 1 in]
              n124 = Delete From Array(array=w234, index=0) -> (deleted portion=w220:dbl, array with subset deleted=w232:dbl[])  [unwired: 1 in]
              n125 = Equal?(x=w219, y=w218) -> (x = y?=w217:bool)
              n126 = Not A Number/Path/Refnum?(number/path/refnum=w219) -> (NaN/Path/Refnum?=w227:bool)
              n127 = Equal?(x=w220, y=w218) -> (x = y?=w216:bool)
              n128 = Not A Number/Path/Refnum?(number/path/refnum=w220) -> (NaN/Path/Refnum?=w228:bool)
              n129 = Or(x=w216, y=w217) -> (x .or. y?=w221:bool)
              n130 = And(x=w228, y=w227) -> (x .and. y?=w226:bool)
              n131 = Select(t=w218, s=w221, f=w223) -> (s? t:f=w225:dbl)
              n132 = Select(t=w222, s=w226, f=w225) -> (s? t:f=w224:dbl)
              n133 = Build Array (concatenate)(w224, w232) -> (w231:dbl[])
            }
            frame "op_13_infix_and" {
              n134 = Delete From Array(array=w257, index=0) -> (deleted portion=w240:dbl, array with subset deleted=w255:dbl[])  [unwired: 1 in]
              n135 = Delete From Array(array=w255, index=0) -> (deleted portion=w241:dbl, array with subset deleted=w253:dbl[])  [unwired: 1 in]
              n136 = Equal?(x=w240, y=w239) -> (x = y?=w238:bool)
              n137 = Not A Number/Path/Refnum?(number/path/refnum=w240) -> (NaN/Path/Refnum?=w248:bool)
              n138 = Equal?(x=w241, y=w239) -> (x = y?=w237:bool)
              n139 = Not A Number/Path/Refnum?(number/path/refnum=w241) -> (NaN/Path/Refnum?=w249:bool)
              n140 = And(x=w237, y=w238) -> (x .and. y?=w242:bool)
              n141 = Or(x=w249, y=w248) -> (x .or. y?=w247:bool)
              n142 = Select(t=w239, s=w242, f=w244) -> (s? t:f=w246:dbl)
              n143 = Select(t=w243, s=w247, f=w246) -> (s? t:f=w245:dbl)
              n144 = Build Array (concatenate)(w245, w253) -> (w252:dbl[])
            }
            frame "op_09_infix_xor" {
              n145 = Delete From Array(array=w276, index=0) -> (deleted portion=w259:dbl, array with subset deleted=w274:dbl[])  [unwired: 1 in]
              n146 = Not A Number/Path/Refnum?(number/path/refnum=w259) -> (NaN/Path/Refnum?=w267:bool)
              n147 = Delete From Array(array=w274, index=0) -> (deleted portion=w258:dbl, array with subset deleted=w272:dbl[])  [unwired: 1 in]
              n148 = Not A Number/Path/Refnum?(number/path/refnum=w258) -> (NaN/Path/Refnum?=w268:bool)
              n149 = Not Equal?(x=w258, y=w259) -> (x != y?=w260:bool)
              n150 = Or(x=w268, y=w267) -> (x .or. y?=w266:bool)
              n151 = Select(t=w261, s=w260, f=w263) -> (s? t:f=w265:dbl)
              n152 = Select(t=w262, s=w266, f=w265) -> (s? t:f=w264:dbl)
              n153 = Build Array (concatenate)(w264, w272) -> (w271:dbl[])
            }
            frame "op_03_prefix_not" {
              n154 = Delete From Array(array=w290, index=0) -> (deleted portion=w281:dbl, array with subset deleted=w283:dbl[])  [unwired: 1 in]
              n155 = Not A Number/Path/Refnum?(number/path/refnum=w281) -> (NaN/Path/Refnum?=w282:bool)
              n156 = Equal?(x=w281, y=w278) -> (x = y?=w280:bool)
              n157 = Select(t=w279, s=w280, f=w278) -> (s? t:f=w277:dbl)
              n158 = Select(t=w284, s=w282, f=w277) -> (s? t:f=w285:dbl)
              n159 = Build Array (concatenate)(w285, w283) -> (w288:dbl[])
            }
            frame "literal_true" {
              n160 = Build Array (concatenate)(w291, w295) -> (w294:dbl[])
            }
            frame "literal_false" {
              n161 = Build Array (concatenate)(w296, w300) -> (w299:dbl[])
            }
            frame "literal_undefined" {
              n162 = Build Array (concatenate)(w301, w305) -> (w304:dbl[])
            }
            frame "literal_decimal" {
              n163 = Scan From String(input string=w309, error in=w308) -> (error out=w307:errorcluster, output 1=w306:dbl)  [unwired: 3 in, 2 out]
              n164 = Build Array (concatenate)(w306, w312) -> (w311:dbl[])
            }
            frame "address_variable" {
              w315 = 1  # remove leading $
              n165 = String Subset(string=w314, offset (0)=w315) -> (substring=w313:string)  [unwired: 1 in]
              n166 = call "FTW-JSON-Object-GetElement-DBL.vi"("JSON Object"=w327, "Key"=w313, "Default Value"=w325, "error in"=w326) -> ("JSON Object out"=w320:refnum<data-value>, "JSON Element Type"=w324:T15, "Value"=w321:dbl, "error out"=w323:errorcluster)  [unwired: 8 in]
              n167 = case shown="\"Not Found\"" w324 {
                tunnel: w323 -> [w330 w333 w337 w340 w343 w346 w356]
                tunnel: [w332 w335 w336 w339 w342 w345 w348] -> w322
                tunnel: w321 -> [w332 w335 w336 w339 w342 w345 _]
                tunnel: w320 -> [w331 w334 w338 w341 w344 w347 w355]
                tunnel: [w331 w334 w338 w341 w344 w347 w354] -> w319
                tunnel: [w330 w333 w337 w340 w343 w346 w353] -> w318
                tunnel: w313 -> [_ _ _ _ _ _ w352]
                tunnel: w317 -> [_ _ _ _ _ _ w351]
                tunnel: w316 -> [_ _ _ _ _ _ w349]
                frame "Not Found" {
                }
                frame "null" {
                }
                frame "Object" {
                }
                frame "Array" {
                }
                frame "String" {
                }
                frame "Number" {
                }
                frame "Boolean" {
                  n168 = call "FTW-JSON-Object-GetElement-Bool.vi"("JSON Object"=w355, "Key"=w352, "error in"=w356) -> ("JSON Object out"=w354:refnum<data-value>, "Value"=w350:bool, "error out"=w353:errorcluster)  [unwired: 9 in, 1 out]
                  n169 = Select(t=w351, s=w350, f=w349) -> (s? t:f=w348:dbl)
                }
              }
              n170 = Build Array (concatenate)(w322, w329) -> (w328:dbl[])
            }
          }
        }
        n171 = call "FTW-JSON-Serialize.vi"("JSON Object"=w76, "error in"=w74) -> ("JSON Object out"=w75:refnum<data-value>, "JSON String (UTF-8)"=w72:string, "error out"=w73:errorcluster)  [unwired: 11 in]
        n172 = Array Size(array=w81) -> (size(s)=w82:i32)
        n173 = call "FTW-JSON-Destroy.vi"("JSON Object"=w75, "error in"=w73) -> ("error out"=w80:errorcluster)  [unwired: 13 in]
        n174 = case shown="Default" w82 {
          selector: w82 -> [w94 _]
          tunnel: w80 -> [w99 w111]
          tunnel: [w98 w112] -> w79
          tunnel: w81 -> [_ w113]
          tunnel: [FTW-Expr-BooleanExpressionResult."inconclusive" ("Result") w109] -> w78
          tunnel: w77 -> [w95 _]
          frame Default {
            n175 = Equal To 0?(x=w94) -> (x = 0?=w96:bool)
            n176 = Empty Array?(array=w95) -> (empty?=w93:bool)
            n177 = And(x=w96, y=w93) -> (x .and. y?=w92:bool)
            n178 = case shown="False" w92 {
              tunnel: w99 -> [w104 w107]
              tunnel: [w103 w106] -> w98
              tunnel: w94 -> [w100 _]
              frame False {
                n179 = Format Into String(format string="Evaluation stack has %d items remaining!" ("Reason this error should never happen"), w100) -> (resulting string=w101:string)  [unwired: 2 in, 1 out]
                n180 = call "FTW-ERR-Assert-DeveloperError.vi"("Reason this error should never happen"=w101, "error in"=w104) -> ("error out"=w103:errorcluster)  [unwired: 13 in]
              }
              frame True {
                n181 = call "FTW-ERR-ThrowInfo.vi"("Informational Message"="Empty expression; no-op.", "error in"=w107) -> ("error out"=w106:errorcluster)  [unwired: 13 in]
              }
            }
          }
          frame 1 {
            n182 = Index Array(array=w113) -> (element=w108:dbl)  [unwired: 1 in]
            n183 = Not A Number/Path/Refnum?(number/path/refnum=w108) -> (NaN/Path/Refnum?=w110:bool)
            n184 = case shown="False" w110 {
              tunnel: [w118 w133] -> w112
              tunnel: w111 -> [w117 w133]
              tunnel: [w115 FTW-Expr-BooleanExpressionResult."inconclusive" ("Result")] -> w109
              tunnel: w108 -> [w114 _]
              frame False {
                n185 = Equal To 0?(x=w114) -> (x = 0?=w116:bool)
                n186 = case shown="False" w116 {
                  tunnel: [w123 w132] -> w118
                  tunnel: w117 -> [w124 w132]
                  tunnel: [w119 FTW-Expr-BooleanExpressionResult."false" ("Result")] -> w115
                  tunnel: w114 -> [w122 _]
                  frame False {
                    n187 = Equal?(x=w122, y=1.0) -> (x = y?=w120:bool)
                    n188 = case shown="False" w120 {
                      tunnel: w124 -> [w127 w129]
                      tunnel: [w126 w129] -> w123
                      tunnel: [FTW-Expr-BooleanExpressionResult."inconclusive" ("Result") FTW-Expr-BooleanExpressionResult."true" ("Result")] -> w119
                      frame False {
                        n189 = call "FTW-ERR-Assert-DeveloperError.vi"("Reason this error should never happen"="Boolean expression evaluated to non-Boolean result!", "error in"=w127) -> ("error out"=w126:errorcluster)  [unwired: 13 in]
                      }
                      frame True {
                      }
                    }
                  }
                  frame True {
                  }
                }
              }
              frame True {
              }
            }
          }
        }
      }
      frame Error {
      }
    }
    n190 = call "FTW-ERR-Assert-DeveloperError.vi"("Reason this error should never happen"="Impossible Error") -> ("error out"=w39:errorcluster)  [unwired: 14 in]
    n191 = Unbundle By Name(w53) -> ("Value Expectation"=w49:T2, "Expression"=w33:string, "Expression Check"=w50:T1, "Expectation"=w48:string)
    n192 = Unbundle By Name(w39) -> ("code"=w37:i32)
    n193 = Unbundle By Name(w25) -> ("code"=w38:i32, "source"=w45:string)
    n194 = Not Equal?(x=w37, y=w38) -> (x != y?=w36:bool)
    n195 = call "FTW-ERR-StatusException.vi"("error to check"=w25) -> ("Exception"=w51:T1)
    n196 = Equal?(x=w51, y=w50) -> (x = y?=w46:bool)
    n197 = Equal?(x=w27, y=w49) -> (x = y?=w47:bool)
    n198 = Compound Arithmetic op=AND(w47, w36, w46) -> (w32:bool)
    n199 = Not(x=w32) -> (.not. x?=w31:bool)
    n200 = Bundle("Expression"=w33, "Expression Check"=w50, "Result"=w27, "Expectation"=w48, w32, "source"=w45, "JSON String (UTF-8)"=w23, "Reverse Polish Notation Token Stack"=w26, w43, "Try Paths"=w29) -> (w54:T16)  [unwired: 1 in]
  }
  "Results" <- w11
  "Array" <- w6
  n201 = And Array Elements(Boolean array=w10) -> (logical AND=w2:bool)
  n202 = call "FTW-Regex-Destroy.vi"("Regex"=w12, "error in"=w7) -> ("error out"=w3:errorcluster)  [unwired: 13 in]
  n203 = call "FTW-ERR-Assert-Truthy.vi"("Assertion"="It works", "Assertion holds true?"=w2, "error in"=w3) -> ("error out"=→"error out":errorcluster)  [unwired: 12 in]
